vi "CheckIP.vi"(11 "port":string) -> (3 "port out":string)   [LabVIEW 2022 SP3]
uses:
  <vilib>/Utility/error.llb/Trim Whitespace One-Sided.vi
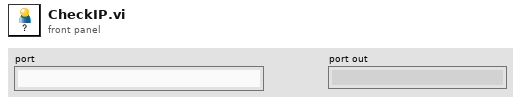
[diagram p1: front panel]
types:
  T1 = cluster{"IP Address":string, "Username":string, "password":string}
  T2 = cluster{"IP Address":string, "Username":string, "password":string}[]
  T3 = cluster{"short name":string, "Full String out":string}[]
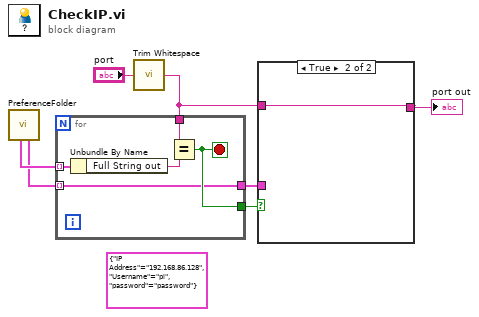
[diagram p0: block diagram]
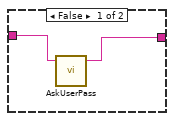
[diagram p2: hidden frame]
diagram:
  (unwired) T1 {"IP Address"="192.168.86.128", "Username"="pi", "password"="password"} ("Raspberry Pi")
  n1 = call "PreferenceFolder.vi"() -> ("SSH Logins"=w6:T2, "Pis"=w7:T3)  [unwired: 5 in, 5 out]
  n2 = call <vilib>:"Trim Whitespace.vi"("string"="port") -> ("trimmed string"=w4:string)  [unwired: 1 in]
  n3 = for {
    tunnel: w4 -> [w12]
    tunnel: [w9] -> w3
    tunnel: [w11] -> w5
    tunnel: w7 -> [w10] mode=indexing
    tunnel: w6 -> [w9] mode=indexing
    stop <- w11 stop-if-true
    n4 = Unbundle By Name(w10) -> ("Full String out"=w8:string)
    n5 = Equal?(x=w12, y=w8) -> (x = y?=w11:bool)
  }
  n6 = case shown="True" w5 {
    tunnel: w4 -> [w14 w15]
    tunnel: w3 -> [_ _]
    tunnel: [w13 w15] -> w1
    frame False {
      n7 = call "AskUserPass.vi"("port"=w14) -> ("Port out"=w13:string)  [unwired: 4 in]
    }
    frame True {
    }
  }
  "port out" <- w1
